vi "CPT-Config.vi"(0 "Cal Stimulus":T2, 5 "Ear":T1=enum."Left", 11 "error in (no error)":errorcluster, 12 "Mic mag graph ref":refnum<vi>) -> (3 "Stimulus waveform":cluster{i32, dbl, dbl[]}, 4 "Stimulus":dbl[](array[numeric]), 6 "Cal Spec Out":T2={"Min Freq (Hz)"=50.0, "Max Freq (Hz)"=50000.0, "Freq Step (Hz)"=50.0, "Waveform"=enum."Chirp", "Attenuation (dB)"=20.0, "Sample Rate (Hz)"=100000.0}, 8 "Mic Avg":dbl[][](array[numeric]), 10 "dt (ms)":dbl, 13 "df (Hz)":dbl, 14 "Cal mic index":i16, 15 "error out":errorcluster)   [LabVIEW 2020]
uses:
  Type Defs/Cal Stimulus.ctl
  epl-vi-lib/Utility VIs/Type Defs/Left-Right ring.ctl
  epl-vi-lib/Connection VIs/Type Defs/Input sources.ctl
  epl-vi-lib/Connection VIs/Type Defs/Output sources.ctl
  epl-vi-lib/PXI DAQ VIs/DAQ Engine VIs/AO Gain and Multiplier VIs/PXI Multipliers to AO Gains (1D).vi
  epl-vi-lib/PXI DAQ VIs/TDT VIs/TDT-Signal Bank Action.ctl
  epl-vi-lib/Utility VIs/Math VIs/dB to Linear (scalar).vi
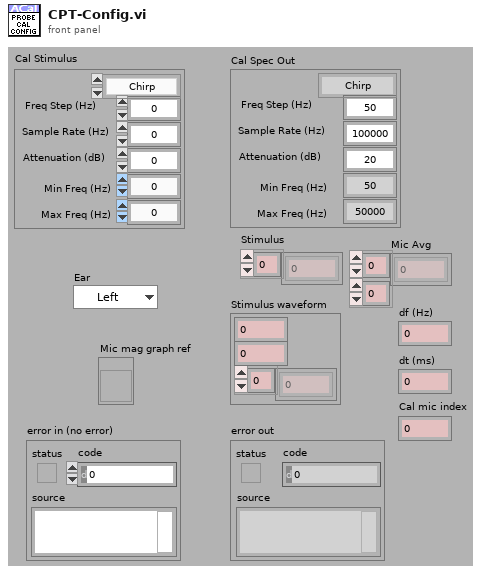
[diagram p1: front panel]
types:
  T1 = typedef "Left-Right ring.ctl" = enum16{"Right", "Left"}
  T2 = typedef "Cal Stimulus.ctl" = cluster{"Min Freq (Hz)":dbl, "Max Freq (Hz)":dbl, "Freq Step (Hz)":dbl, "Waveform":enum16{"Chirp", "Weighted"}, "Attenuation (dB)":dbl, "Sample Rate (Hz)":dbl}
  T3 = typedef "TDT-Signal Bank Action.ctl" = enum16{"Init", "Write", "Read", "Rewrite", "Reset", "Recycle", "Ramp up", "Ramp down", "Zero"}
  T4 = typedef "Input sources.ctl" = u16
  T5 = typedef "Output sources.ctl" = u16
  T6 = typedef "TDT-Device Config.ctl" = cluster{"Output":T7, "Input":T9}
  T7 = typedef "TDT-Output source.ctl" = cluster{"Device":T8, "Num":i32}
  T8 = typedef "TDT-Device ID.ctl" = enum16{"None", "PA5", "RP2", "RL2", "RA16", "RV8", "RX5", "RX6", "RX7", "RX8", "RZ2", "RZ5", "RZ6"}
  T9 = typedef "TDT-Input source.ctl" = enum16{"Front Panel", "RA4LI", "RA16LI"}
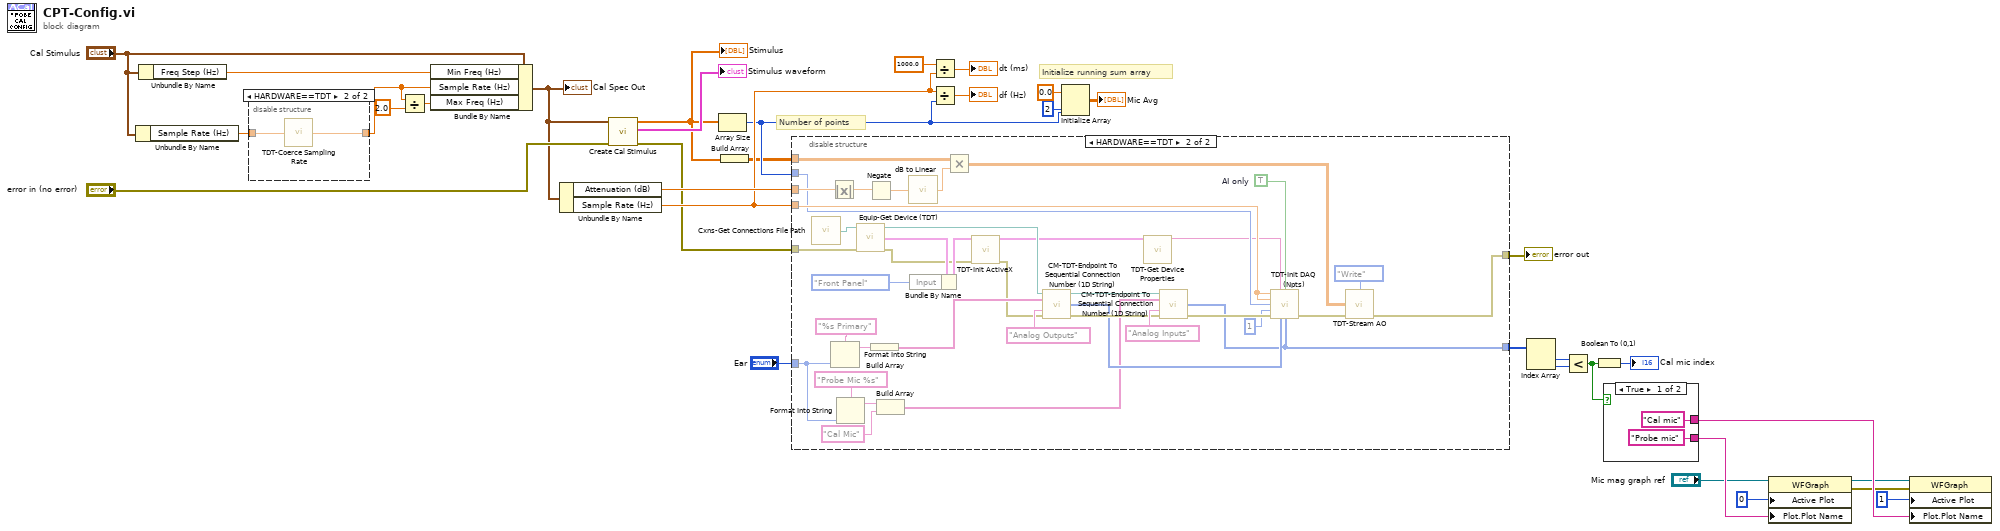
[diagram p0: block diagram]
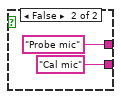
[diagram p2: hidden frame]
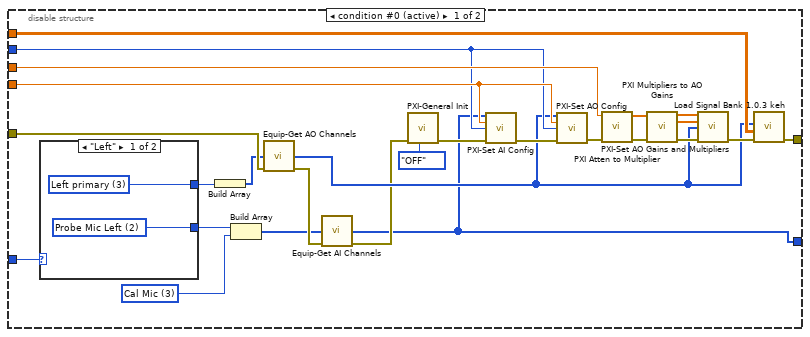
[diagram p4: hidden frame]
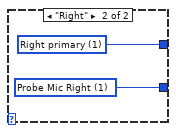
[diagram p5: hidden frame]
diagram:
  # "Number of points"
  # "Initialize running sum array"
  n1 = Unbundle By Name("Cal Stimulus") -> ("Sample Rate (Hz)"=w15:dbl)
  n2 = Unbundle By Name("Cal Stimulus") -> ("Freq Step (Hz)"=w21:dbl)
  n3 = disable-structure shown="HARDWARE==TDT" {
    disable-tunnel: [w36 w38] -> w1
    disable-tunnel: w15 -> [w36 w37]
    frame condition #0 (active) {
    }
    frame condition #1 {
      n4 = call "TDT-Coerce Sampling Rate.vi"("Fs (Hz)"=w37) -> ("Coerced"=w38:dbl)
    }
  }
  n5 = Divide(x=w1, y=2.0) -> (x/y=w20:dbl)
  n6 = Bundle By Name(cluster="Cal Stimulus", "Min Freq (Hz)"=w21, "Sample Rate (Hz)"=w1, "Max Freq (Hz)"=w20) -> (w17:T2)
  "Cal Spec Out" <- w17
  n7 = Unbundle By Name(w17) -> ("Attenuation (dB)"=w33:dbl, "Sample Rate (Hz)"=w24:dbl)
  n8 = call "Create Cal Stimulus.vi"("error in (no error)"="error in (no error)", "Cal Stimulus"=w17) -> ("error out"=w18:errorcluster, "Stimulus waveform"=→"Stimulus waveform":cluster{i32, dbl, dbl[]}, "Stimulus"=w34:dbl[])  [unwired: 7 in]
  "Stimulus" <- w34
  n9 = Array Size(array=w34) -> (size(s)=w23:i32)
  n10 = Build Array(w34) -> (w22:dbl[][])
  n11 = disable-structure shown="HARDWARE==TDT" {
    disable-tunnel: w33 -> [w62 w100]
    disable-tunnel: [w61 w97] -> w25
    disable-tunnel: w24 -> [w54 w90]
    disable-tunnel: w23 -> [w53 w88]
    disable-tunnel: w22 -> [w51 w96]
    disable-tunnel: w18 -> [w48 w86]
    disable-tunnel: "Ear" -> [w46 w76]
    disable-tunnel: [w39 w73] -> w3
    frame condition #0 (active) {
      w40 = T4 3 items=["--unused--", "Probe Mic Right", "Probe Mic Left", "Cal Mic", "ABR", "CAP Right", "CAP Left", "Startle piezo", "Temperature", "Heart rate", "Accelerometer", "Startle piezo 2"] ("element")
      n12 = case shown="\"Left\"" w46 {
        tunnel: [w66 w68] -> w42
        tunnel: [w65 w67] -> w41
        frame "Left" {
          w66 = T5 3 items=["--unused--", "Right primary", "Right secondary", "Left primary", "Left secondary", "Shocks", "Startle", "Background"] ("Ring")
          w65 = T4 2 items=["--unused--", "Probe Mic Right", "Probe Mic Left", "Cal Mic", "ABR", "CAP Right", "CAP Left", "Startle piezo", "Temperature", "Heart rate"] ("Ring")
        }
        frame "Right" {
          w68 = T5 1 items=["--unused--", "Right primary", "Right secondary", "Left primary", "Left secondary", "Shocks", "Startle", "Background"] ("Ring")
          w67 = T4 1 items=["--unused--", "Probe Mic Right", "Probe Mic Left", "Cal Mic", "ABR", "CAP Right", "CAP Left", "Startle piezo", "Temperature", "Heart rate"] ("Ring")
        }
      }
      n13 = Build Array(w42) -> (w43:T5[])
      n14 = Build Array(w41, w40) -> (w44:T4[])
      n15 = call "Equip-Get AO Channels.vi"("Outputs"=w43, "error in (no error)"=w48) -> ("AO Channels"=w49:i32[], "error out"=w45:errorcluster)  [unwired: 12 in]
      n16 = call "Equip-Get AI Channels.vi"("Inputs"=w44, "error in (no error)"=w45) -> ("AI Channels"=w39:i32[], "error out"=w47:errorcluster)  [unwired: 12 in]
      n17 = call "PXI-General Init.vi"("Double Buffer Mode"=enum32{"OFF", "ENABLED", "FORCED"}."OFF", "error in (no error)"=w47) -> ("error out"=w57:errorcluster)  [unwired: 9 in]
      n18 = call "PXI-Set AI Config.vi"("AI Channels"=w39, "Sampling Rate (Hz)"=w54, "Buffer Size"=w53, "error in (no error)"=w57) -> ("error out"=w55:errorcluster)  [unwired: 11 in]
      n19 = call "PXI-Set AO Config.vi"("AO Channels"=w49, "Sampling Rate (Hz)"=w54, "Buffer Size"=w53, "error in (no error)"=w55) -> ("error out"=w56:errorcluster)  [unwired: 11 in]
      n20 = call "PXI Atten to Multiplier.vi"("error in (no error)"=w56, "Attenuation"=w62) -> ("error out"=w64:errorcluster, "Multiplier setting"=w63:dbl[])  [unwired: 8 in]
      n21 = call-poly "PXI Multipliers to AO Gains.vi"("Multipliers in"=w63, "error in (no error)"=w64) -> ("Multipliers out"=w59:dbl[], "Gains"=w58:dbl[], "error out"=w60:errorcluster)  [unwired: 11 in]
      n22 = call "PXI-Set AO Gains and Multipliers.vi"("Multipliers"=w59, "Gains"=w58, "AO Channels"=w49, "error in (no error)"=w60) -> ("error out"=w52:errorcluster)  [unwired: 11 in]
      n23 = call "Load Signal Bank 1.0.3 keh.vi"("error in (no error)"=w52, "Input array"=w51, "Active AO Array"=w49) -> ("error out"=w61:errorcluster)  [unwired: 6 in, 2 out]
    }
    frame condition #1 {
      w92 = TRUE  # AI only
      n24 = call "Cxns-Get Connections File Path.vi"() -> ("Path Out"=w87:path)  [unwired: 1 in]
      n25 = Absolute Value(x=w100) -> (abs(x)=w99:dbl)
      n26 = Format Into String(format string="%s Primary", w76) -> (resulting string=w80:string)  [unwired: 2 in, 1 out]
      n27 = Format Into String(format string="Probe Mic %s", w76) -> (resulting string=w77:string)  [unwired: 2 in, 1 out]
      n28 = call "Equip-Get Device (TDT).vi"("Path In"=w87, "error in (no error)"=w86) -> ("Path Out"=w83:path, "TDT-Device Config"=w84:T6, "error out"=w71:errorcluster)  [unwired: 11 in]
      n29 = Negate(x=w99) -> (-x=w101:dbl)
      n30 = Build Array(w80) -> (w79:string[])
      n31 = Build Array(w77, "Cal Mic" ("String")) -> (w74:string[])
      n32 = call-poly "dB to Linear.vi"("dB"=w101) -> ("linear"=w95:dbl)
      n33 = Bundle By Name(cluster=w84, "Input"=enum16{"Front Panel", "RA4LI", "RA16LI"}."Front Panel") -> (w72:T6)
      n34 = Multiply(x=w96, y=w95) -> (x*y=w94:dbl[][])
      n35 = call "TDT-Init ActiveX.vi"("TDT-Device Config"=w72, "error in (no error)"=w71) -> ("TDT-Device Config out"=w70:T6, "error out"=w69:errorcluster)  [unwired: 10 in, 2 out]
      n36 = call "CM-TDT-Endpoint To Sequential Connection Number (1D String).vi"("Path In"=w83, "Endpoints"=w79, "Section"="Analog Outputs", "error in (no error)"=w69) -> ("Path Out"=w105:path, "SeqCxnNum"=w91:i32[], "error out"=w104:errorcluster)  [unwired: 9 in]
      n37 = call "TDT-Get Device Properties.vi"("TDT-Device Config"=w70) -> ("Circuit File"=w82:string)  [unwired: 9 in, 5 out]
      n38 = call "CM-TDT-Endpoint To Sequential Connection Number (1D String).vi"("Path In"=w105, "Endpoints"=w74, "Section"="Analog Inputs", "error in (no error)"=w104) -> ("SeqCxnNum"=w73:i32[], "error out"=w93:errorcluster)  [unwired: 9 in, 1 out]
      n39 = call "TDT-Init DAQ (Npts).vi"("AO Fs (Hz)"=w90, "Circuit"=w82, "AI only"=w92, "AI Fs (Hz)"=w90, "Num AO Pts"=w88, "Num AO Buffers"=1, "error in (no error)"=w93, "AO Channels"=w91, "AI Channels"=w73) -> ("error out"=w98:errorcluster)  [unwired: 2 in, 4 out]
      n40 = call "TDT-Stream AO.vi"("Action"=TDT-Signal_Bank_Action."Write", "Output array"=w94, "error in (no error)"=w98) -> ("error out"=w97:errorcluster)  [unwired: 12 in]
    }
  }
  "error out" <- w25
  n41 = Divide(x=1000.0, y=w24) -> (x/y=→"dt (ms)":dbl)
  n42 = Divide(x=w24, y=w23) -> (x/y=→"df (Hz)":dbl)
  n43 = Initialize Array(0.0 ("element"), 2 ("dimension size"), w23) -> (→"Mic Avg":dbl[][])
  n44 = Index Array(array=w3) -> (element #1=w12:i32, element #2=w13:i32)  [unwired: 2 in]
  n45 = Less?(x=w12, y=w13) -> (x < y?=w5:bool)
  n46 = Boolean To (0,1)(Boolean=w5) -> (0, 1=→"Cal mic index":i16)
  n47 = case shown="True" w5 {
    tunnel: ["Cal mic" "Probe mic"] -> w10
    tunnel: ["Probe mic" "Cal mic"] -> w11
    frame True {
    }
    frame False {
    }
  }
  n48 = property class="WFGraph"(reference="Mic mag graph ref", "Active Plot"=u32 0, "Plot.Plot Name"=w11) -> (reference out=w7:refnum<vi>, error out=w8:errorcluster)  [unwired: 1 in]
  n49 = property class="WFGraph"(reference=w7, error in=w8, "Active Plot"=u32 1, "Plot.Plot Name"=w10) -> ()  [unwired: 2 out]
